vi "Motor_Control.vi"(10 "Stage_Motor":T1=enum."Off", 11 "Intake_Motor":T1=enum."Off") -> (2 "Stage_Motor_CMD":dbl, 3 "Intake_Motor_CMD":dbl)   [LabVIEW 2015]
uses:
  Motor_Dir_Type_Def.ctl
panel:
  in  "Stage_Off":dbl format="%#_13g"
  in  "Intake_Off":dbl format="%#_13g"
  in  "In_Stage":dbl=1.0
  in  "Out_Stage":dbl=-1.0
  in  "In_Intake":dbl=1.0
  in  "Out_Intake":dbl=-1.0
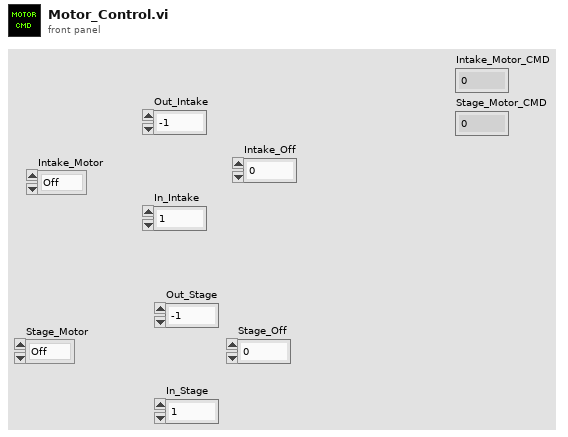
[diagram p1: front panel]
types:
  T1 = typedef "Motor_Dir_Type_Def.ctl" = enum16{"In", "Out", "Off"}
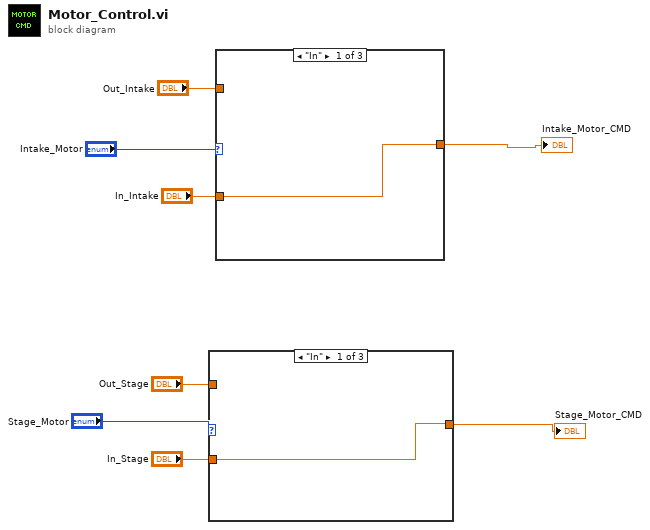
[diagram p0: block diagram]
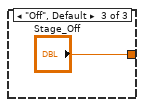
[diagram p3: hidden frame]
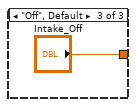
[diagram p5: hidden frame]
diagram:
  n1 = case shown="\"In\"" "Stage_Motor" {
    tunnel: "Out_Stage" -> [_ w10 _]
    tunnel: "In_Stage" -> [w9 _ _]
    tunnel: [w9 w10 "Stage_Off"] -> w1
    frame "In" {
    }
    frame "Out" {
    }
    frame "Off", Default {
    }
  }
  "Stage_Motor_CMD" <- w1
  n2 = case shown="\"In\"" "Intake_Motor" {
    tunnel: "Out_Intake" -> [_ w13 _]
    tunnel: "In_Intake" -> [w12 _ _]
    tunnel: [w12 w13 "Intake_Off"] -> w2
    frame "In" {
    }
    frame "Out" {
    }
    frame "Off", Default {
    }
  }
  "Intake_Motor_CMD" <- w2
